vi "Registration.vi"(8 "error in (no error)":errorcluster, 10 "Message":refnum<class "MSG.lvclass">, 11 "ObserverRegistry in":refnum<class "ObserverRegistry.lvclass">) -> (0 "error out":errorcluster, 2 "Message (Register Commands filtered out)":refnum<class "MSG.lvclass">, 3 "ObserverRegistry out":refnum<class "ObserverRegistry.lvclass">)   [LabVIEW 2011, in "Messenging.lvlib" / "ObserverRegistry.lvclass"]
doc: "Inspects a Message and acts on it if it is an Observer Registry Command (and outputs an empty message). Otherwise passes the message through unchanged."
uses:
  ObserverRegistry.lvclass
  Commands/ParentCommand/ObserverRegistryCommand.lvclass
  Interprocess Messenger/TextVarientMessage/MSG.lvclass
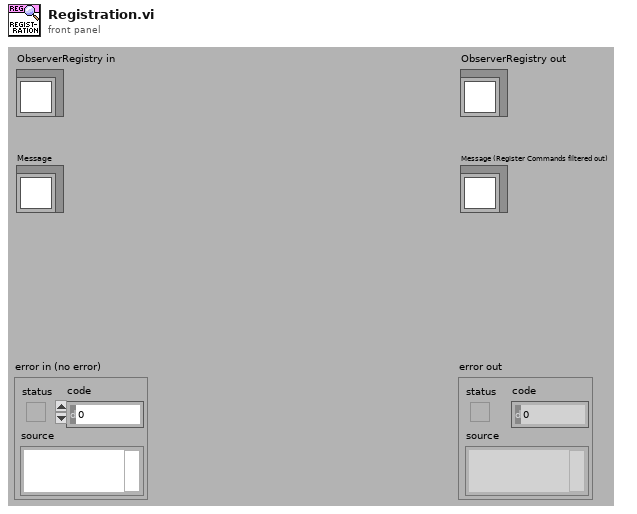
[diagram p1: front panel]
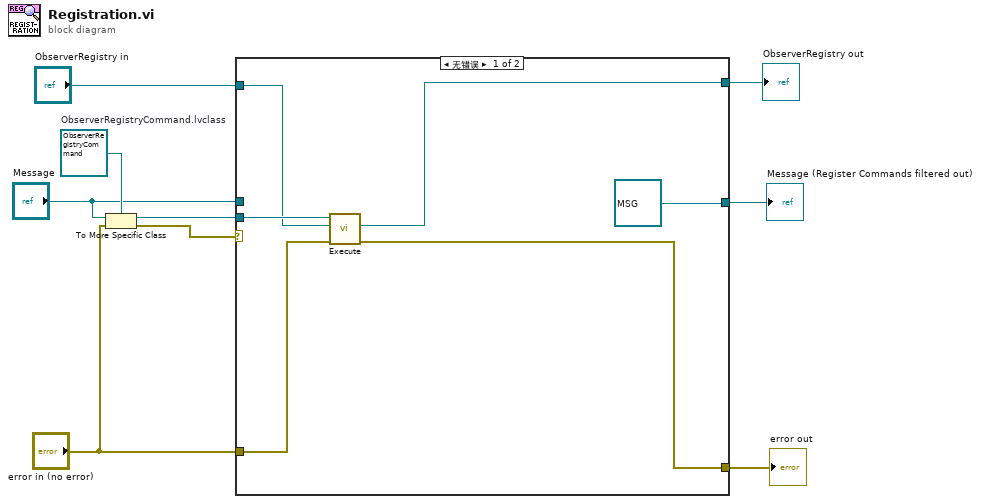
[diagram p0: block diagram]
diagram:
  w6 = refnum<class "ObserverRegistryCommand.lvclass"> refnum  # ObserverRegistryCommand.lvclass
  n1 = To More Specific Class(target class=w6, reference="Message", error in="error in (no error)") -> (specific class reference=w4:refnum<class "ObserverRegistryCommand.lvclass">, error out=w5:errorcluster)
  n2 = case shown="无错误" w5 {
    tunnel: "ObserverRegistry in" -> [w14 w18]
    tunnel: [w13 w18] -> w8
    tunnel: [w11 w16] -> w7
    tunnel: w4 -> [w15 _]
    tunnel: "Message" -> [_ w17]
    tunnel: [refnum<class "MSG.lvclass"> refnum ("Message") w17] -> w2
    tunnel: "error in (no error)" -> [w12 w16]
    frame No Error {
      n3 = call-dynamic "Execute.vi"("error in (no error)"=w12, "ObserverRegistry in"=w14, "ObserverRegistryCommand"=w15) -> ("error out"=w11:errorcluster, "ObserverRegistry out"=w13:refnum<class "ObserverRegistry.lvclass">)  [unwired: 7 out]
    }
    frame Error {
      # "Not an ObserverRegister Command, so ignore it"
    }
  }
  "error out" <- w7
  "ObserverRegistry out" <- w8
  "Message (Register Commands filtered out)" <- w2
